vi "Punto_desplazado_i.vi"(10 "Numeric":dbl, 11 "Array out":dbl[](array[numeric])) -> (3 "Array":dbl[](array[numeric]))   [LabVIEW 2011]
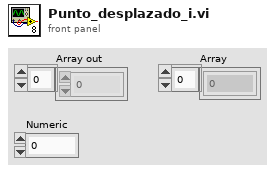
[diagram p1: front panel]
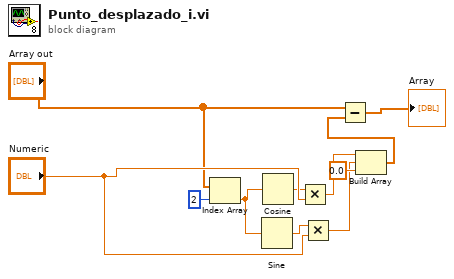
[diagram p0: block diagram]
diagram:
  n1 = Index Array(array="Array out", index=2) -> (element=w10:dbl)
  n2 = Sine(x=w10) -> (sin(x)=w1:dbl)
  n3 = Cosine(x=w10) -> (cos(x)=w2:dbl)
  n4 = Multiply(x=w2, y="Numeric") -> (x*y=w4:dbl)
  n5 = Multiply(x=w1, y="Numeric") -> (x*y=w5:dbl)
  n6 = Build Array(w4, w5, 0.0 ("element")) -> (w7:dbl[])
  n7 = Subtract(x="Array out", y=w7) -> (x-y=→"Array":dbl[])
